vi "Obtain Hwnd and instantiate.vi"(0 "Py Doc in":refnum<class "Py Doc.lvclass">, 11 "error in (no error)":errorcluster) -> (4 "Document Out":refnum<class "Document.lvclass">, 6 "Document out":refnum<class "Document.lvclass">, 15 "error out":errorcluster)   [LabVIEW 2016, in "Py Doc.lvclass"]
uses:
  Py Doc.lvclass
  D:/MDI Project/source code/Document/Document.lvclass
  Document.lvclass
  Document.lvclass/Document.ctl
  Child Classes/Py Editor/Py Editor.lvclass
  Child Classes/Py Shell/Py Shell.lvclass
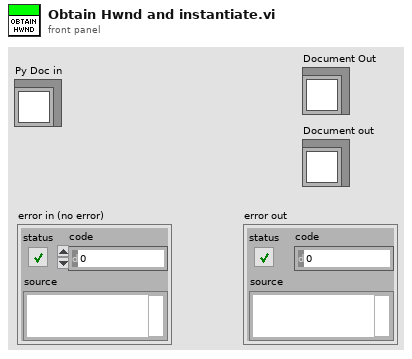
[diagram p1: front panel]
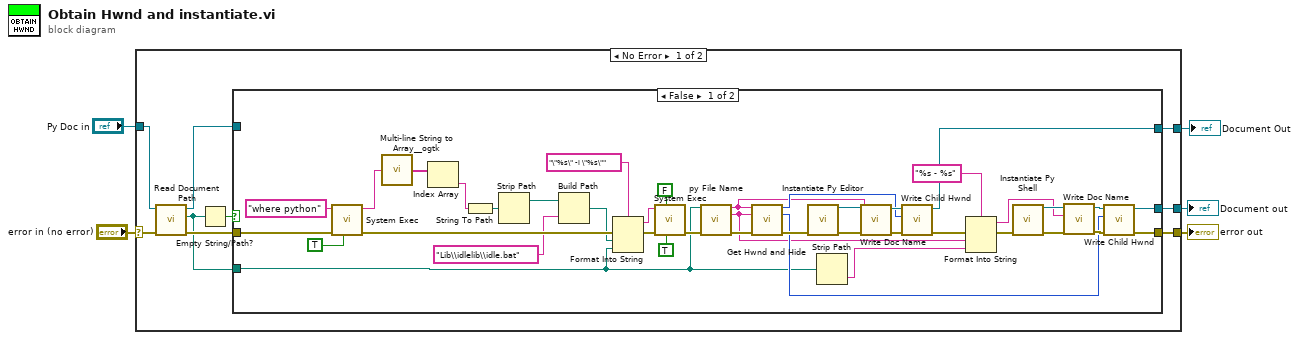
[diagram p0: block diagram]
diagram:
  n1 = case shown="No Error" "error in (no error)" {
    selector: "error in (no error)" -> [w13 w58]
    tunnel: "Py Doc in" -> [w11 w57]
    tunnel: [w14 w58] -> w4
    tunnel: [w7 w57] -> w2
    tunnel: [w6 w57] -> w1
    frame No Error {
      n2 = call "Read Document Path.vi"("error in (no error)"=w13, "Document in"=w11) -> ("error out"=w12:errorcluster, "Document Path"=w9:path, "Document out"=w10:refnum<class "Py Doc.lvclass">)  [unwired: 7 in]
      n3 = Empty String/Path?(string/path=w9) -> (empty?=w8:bool)
      n4 = case shown="False" w8 {
        tunnel: [w24 w56] -> w14
        tunnel: w12 -> [w37 w56]
        tunnel: w10 -> [_ w55]
        tunnel: w9 -> [w20 _]
        tunnel: [w22 w55] -> w7
        tunnel: [w21 w55] -> w6
        frame False {
          n5 = call <vilib>:"System Exec.vi"("run minimized? (F)"=TRUE, "error in (no error)"=w37, "command line"="where python") -> ("error out"=w54:errorcluster, "standard output"=w35:string)  [unwired: 5 in, 2 out]
          n6 = call <userlib>:"Multi-line String to Array__ogtk.vi"("string"=w35) -> ("lines"=w36:string[])
          n7 = Index Array(array=w36) -> (element=w34:string)  [unwired: 1 in]
          n8 = String To Path(string=w34) -> (path=w50:path)
          n9 = Strip Path(path=w50) -> (stripped path=w51:path)  [unwired: 1 out]
          n10 = Build Path(base path=w51, name or relative path="Lib\\idlelib\\idle.bat") -> (appended path=w53:path)
          n11 = Format Into String(format string="\"%s\" -i \"%s\"", error in=w54, w53, w20) -> (resulting string=w39:string, error out=w38:errorcluster)  [unwired: 1 in]
          n12 = call <vilib>:"System Exec.vi"("run minimized? (F)"=TRUE, "wait until completion? (T)"=FALSE, "error in (no error)"=w38, "command line"=w39) -> ("error out"=w44:errorcluster)  [unwired: 4 in, 3 out]
          n13 = call "py File Name.vi"("Path"=w20, "error in (no error)"=w44) -> ("Doc Name"=w45:string, "Shell Name"=w17:string, "error out"=w42:errorcluster)  [unwired: 11 in]
          n14 = call "Get Hwnd and Hide.vi"("Doc Name"=w45, "Shell Name"=w17, "error in (no error)"=w42) -> ("Child hwnd"=w46:u32, "Shell hwnd"=w23:u32, "error out"=w30:errorcluster)  [unwired: 10 in]
          n15 = call "Instantiate Py Editor.vi"("error in (no error)"=w30) -> ("Document.lvclass"=w28:refnum<class "Document.lvclass">, "error out"=w29:errorcluster)  [unwired: 13 in]
          n16 = Strip Path(path=w20) -> (name=w16:string)  [unwired: 1 out]
          n17 = call "Write Doc Name.vi"("error in (no error)"=w29, "Doc Name"=w45, "Document in"=w28) -> ("error out"=w48:errorcluster, "Document out"=w47:refnum<class "Document.lvclass">)  [unwired: 7 in]
          n18 = call "Write Child Hwnd.vi"("error in (no error)"=w48, "Child Hwnd"=w46, "Document in"=w47) -> ("error out"=w25:errorcluster, "Document out"=w21:refnum<class "Document.lvclass">)  [unwired: 7 in]
          n19 = Format Into String(format string="%s - %s", error in=w25, w17, w16) -> (resulting string=w18:string, error out=w19:errorcluster)  [unwired: 1 in]
          n20 = call "Instantiate Py Shell.vi"("error in (no error)"=w19) -> ("Document.lvclass"=w31:refnum<class "Document.lvclass">, "error out"=w27:errorcluster)  [unwired: 13 in]
          n21 = call "Write Doc Name.vi"("error in (no error)"=w27, "Doc Name"=w18, "Document in"=w31) -> ("error out"=w26:errorcluster, "Document out"=w32:refnum<class "Document.lvclass">)  [unwired: 7 in]
          n22 = call "Write Child Hwnd.vi"("error in (no error)"=w26, "Child Hwnd"=w23, "Document in"=w32) -> ("error out"=w24:errorcluster, "Document out"=w22:refnum<class "Document.lvclass">)  [unwired: 7 in]
        }
        frame True {
        }
      }
    }
    frame Error {
    }
  }
  "error out" <- w4
  "Document out" <- w2
  "Document Out" <- w1
